vi "sv_Audio Frequency Weighting.vi"(1 "spectrum type":enum16{"Power", "Amplitude"}(ring), 2 "dB On (T)":bool=TRUE, 3 "frequency [Hz]":dbl=1000.0 min=0.0 format="%.2f", 4 "weighting filter":T1 items=["Linear", "A-weighting", "B-weighting", "C-weighting", "ITU-R 468-4", "Dolby", "CCITT", "C-message", "Wb", "Wc", "Wd", "We", "Wf", "Wh", "Wj", "Wk", "Wm", "AES17 20 kHz lowpass", "AES17 40 kHz lowpass", "AES17 20 kHz highpass", "AES17 40 kHz highpass"]) -> (0 "relative response level":dbl format="%.2e")   [LabVIEW 2017]
uses:
  <vilib>/addons/_NISVFA/_Shared subVIs/Controls/svc_Weighting Filter Text Ring.ctl
  <vilib>/Analysis/NI_AALPro.lvlib
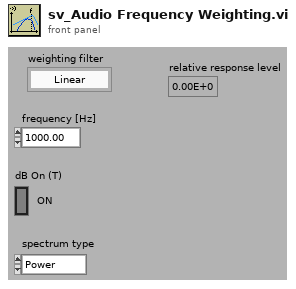
[diagram p1: front panel]
types:
  T1 = typedef "svc_Weighting Filter Text Ring.ctl" = u16
  T2 = cluster{"log(frequency)":dbl[], "response [dB]":dbl[]}
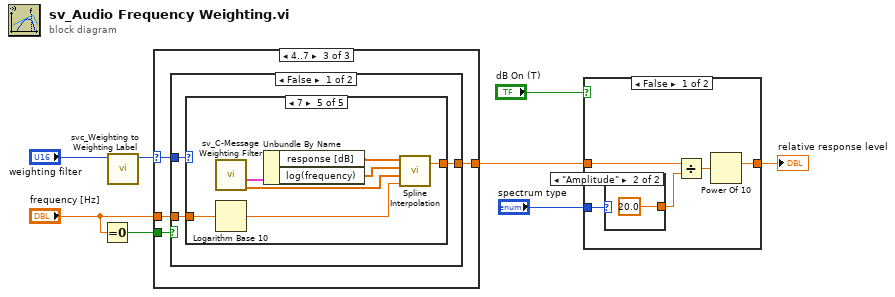
[diagram p0: block diagram]
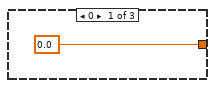
[diagram p2: hidden frame]
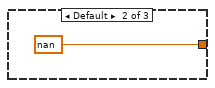
[diagram p3: hidden frame]
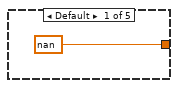
[diagram p4: hidden frame]
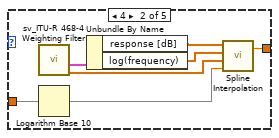
[diagram p5: hidden frame]
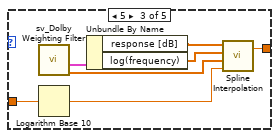
[diagram p6: hidden frame]
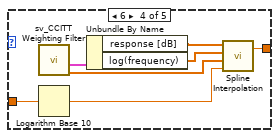
[diagram p7: hidden frame]
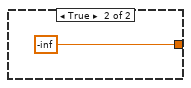
[diagram p8: hidden frame]
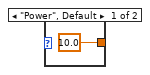
[diagram p9: hidden frame]
diagram:
  n1 = Equal To 0?(x="frequency [Hz]") -> (x = 0?=w2:bool)
  n2 = call <vilib>:"svc_Weighting to Weighting Label.vi"("weighting filter"="weighting filter") -> ("weighting enum"=w1:T1)  [unwired: 9 in, 1 out]
  n3 = case shown="4..7" w1 {
    selector: w1 -> [_ _ w11]
    tunnel: [0.0 nan w14] -> w6
    tunnel: "frequency [Hz]" -> [_ _ w13]
    tunnel: w2 -> [_ _ w12]
    frame 0 {
    }
    frame Default {
    }
    frame 4..7 {
      n4 = case shown="False" w12 {
        tunnel: [w17 -inf] -> w14
        tunnel: w11 -> [w16 _]
        tunnel: w13 -> [w15 _]
        frame False {
          n5 = case shown="7" w16 {
            tunnel: [nan w20 w27 w34 w41] -> w17
            tunnel: w15 -> [_ w19 w26 w33 w40]
            frame Default {
            }
            frame 4 {
              n6 = call <vilib>:"sv_ITU-R 468-4 Weighting Filter.vi"() -> ("ITU-R 468-4 interpolant (log scale)"=w23:dbl[], "ITU-R 468-4 relative response"=w22:T2)  [unwired: 8 in, 2 out]
              n7 = Logarithm Base 10(1:w19) -> (0:w21:dbl)
              n8 = Unbundle By Name(w22) -> ("response [dB]"=w25:dbl[], "log(frequency)"=w24:dbl[])
              n9 = call <vilib>:"Spline Interpolation.vi"("x value"=w21, "Interpolant"=w23, "X"=w24, "Y"=w25) -> ("interpolation value"=w20:dbl)  [unwired: 1 out]
            }
            frame 5 {
              n10 = call <vilib>:"sv_Dolby Weighting Filter.vi"() -> ("Dolby interpolant (log scale)"=w30:dbl[], "Dolby relative response"=w29:T2)  [unwired: 8 in, 2 out]
              n11 = Logarithm Base 10(1:w26) -> (0:w28:dbl)
              n12 = Unbundle By Name(w29) -> ("response [dB]"=w32:dbl[], "log(frequency)"=w31:dbl[])
              n13 = call <vilib>:"Spline Interpolation.vi"("x value"=w28, "Interpolant"=w30, "X"=w31, "Y"=w32) -> ("interpolation value"=w27:dbl)  [unwired: 1 out]
            }
            frame 6 {
              n14 = call <vilib>:"sv_CCITT Weighting Filter.vi"() -> ("CCITT interpolant"=w37:dbl[], "CCITT relative response"=w36:T2)  [unwired: 8 in, 2 out]
              n15 = Logarithm Base 10(1:w33) -> (0:w35:dbl)
              n16 = Unbundle By Name(w36) -> ("response [dB]"=w39:dbl[], "log(frequency)"=w38:dbl[])
              n17 = call <vilib>:"Spline Interpolation.vi"("x value"=w35, "Interpolant"=w37, "X"=w38, "Y"=w39) -> ("interpolation value"=w34:dbl)  [unwired: 1 out]
            }
            frame 7 {
              n18 = call <vilib>:"sv_C-Message Weighting Filter.vi"() -> ("C-message interpolant (log scale)"=w44:dbl[], "C-message relative response"=w43:T2)  [unwired: 8 in, 2 out]
              n19 = Logarithm Base 10(1:w40) -> (0:w42:dbl)
              n20 = Unbundle By Name(w43) -> ("response [dB]"=w46:dbl[], "log(frequency)"=w45:dbl[])
              n21 = call <vilib>:"Spline Interpolation.vi"("x value"=w42, "Interpolant"=w44, "X"=w45, "Y"=w46) -> ("interpolation value"=w41:dbl)  [unwired: 1 out]
            }
          }
        }
        frame True {
        }
      }
    }
  }
  n22 = case shown="False" "dB On (T)" {
    tunnel: w6 -> [w50 w55]
    tunnel: [w48 w55] -> w7
    tunnel: "spectrum type" -> [w52 _]
    frame False {
      n23 = case shown="\"Amplitude\"" w52 {
        tunnel: [10.0 ("interpolation value") 20.0 ("interpolation value")] -> w51
        frame "Power", Default {
        }
        frame "Amplitude" {
        }
      }
      n24 = Divide(x=w50, y=w51) -> (x/y=w49:dbl)
      n25 = Power Of 10(x=w49) -> (10^x=w48:dbl)
    }
    frame True {
    }
  }
  "relative response level" <- w7
